vi "demux1_10(x6)_encode.vi"(8 "error in (no error)":errorcluster, 10 "demux1_10(x6)_encode":T1(ring), 11 "Mem_mapping in":u16[](array[numeric])) -> (0 "error out":errorcluster, 3 "MemMapping Out":u16[](array[numeric]))   [LabVIEW 2018, in "MB Relay.lvlib"]
uses:
  MB Relay.lvlib
panel:
  out "demux10_1(x6)":u16[](array[numeric])
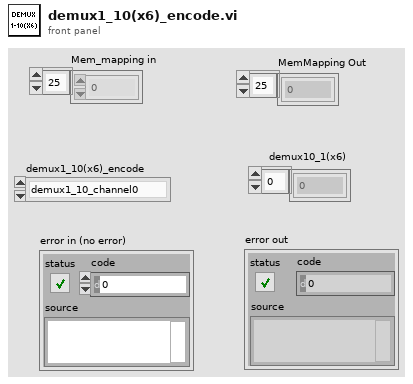
[diagram p1: front panel]
types:
  T1 = enum16{"demux1_10_channel0", "demux1_10_channel1", "demux1_10_channel2", "demux1_10_channel3", "demux1_10_channel4", "demux1_10_channel5", "demux1_10_channel6", "demux1_10_channel7", "demux1_10_channel8", "demux1_10_channel9", "demux1_10_channel10"}
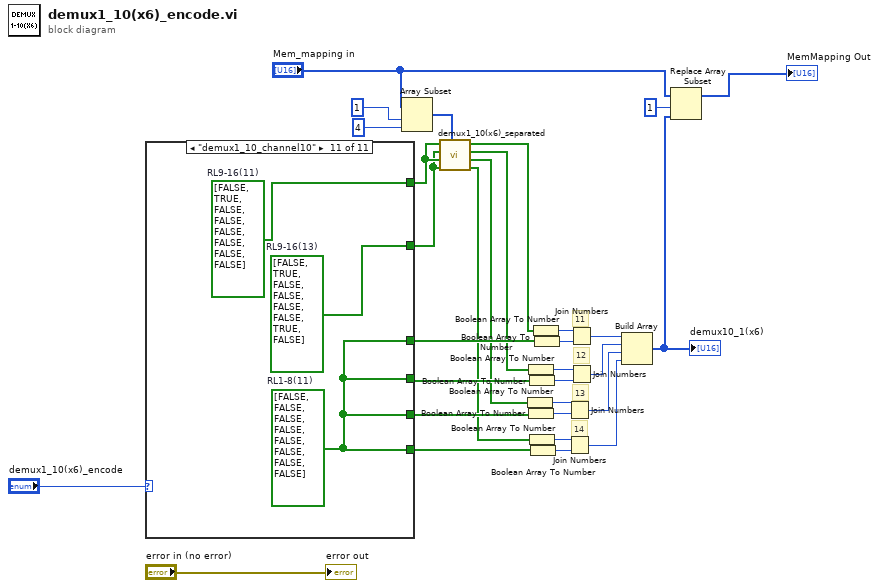
[diagram p0: block diagram]
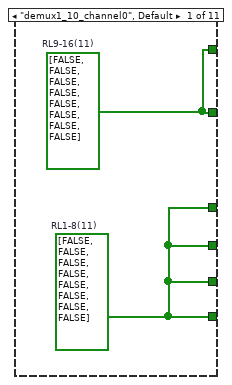
[diagram p2: hidden frame]
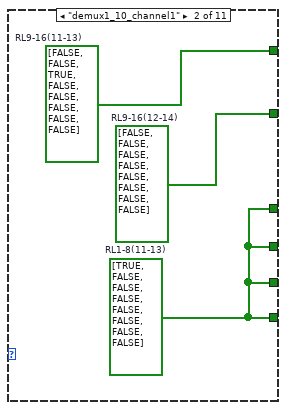
[diagram p3: hidden frame]
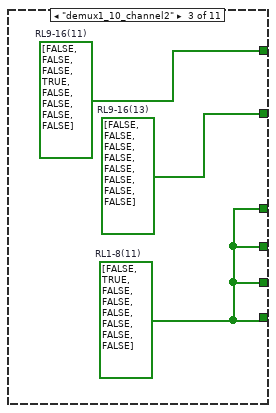
[diagram p4: hidden frame]
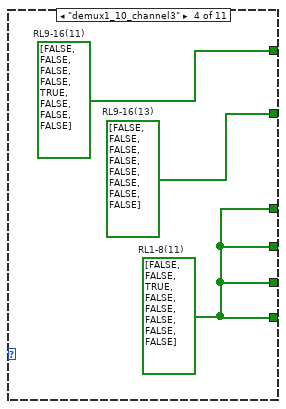
[diagram p5: hidden frame]
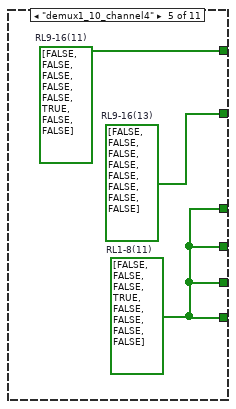
[diagram p6: hidden frame]
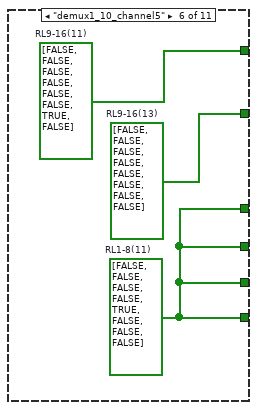
[diagram p7: hidden frame]
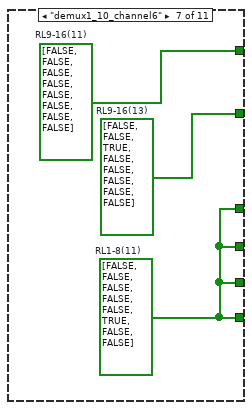
[diagram p8: hidden frame]
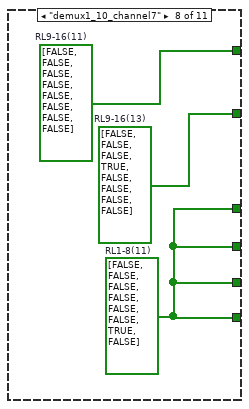
[diagram p9: hidden frame]
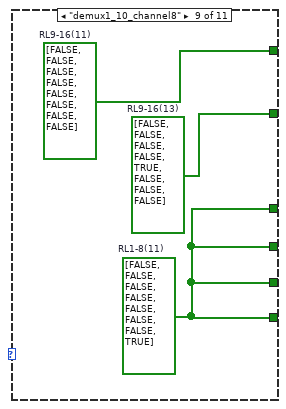
[diagram p10: hidden frame]
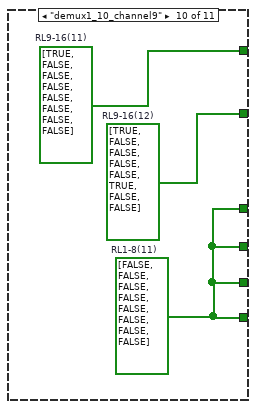
[diagram p11: hidden frame]
diagram:
  # "14"
  # "13"
  # "12"
  # "11"
  n1 = case shown="\"demux1_10_channel10\"" "demux1_10(x6)_encode" {
    tunnel: [w33 w36 w39 w42 w45 w48 w51 w54 w57 w60 w63] -> w18
    tunnel: [w33 w36 w39 w42 w45 w48 w51 w54 w57 w60 w63] -> w19
    tunnel: [w33 w36 w39 w42 w45 w48 w51 w54 w57 w60 w63] -> w17
    tunnel: [w33 w36 w39 w42 w45 w48 w51 w54 w57 w60 w63] -> w22
    tunnel: [w32 w35 w38 w41 w44 w47 w50 w53 w56 w59 w62] -> w2
    tunnel: [w32 w34 w37 w40 w43 w46 w49 w52 w55 w58 w61] -> w1
    frame "demux1_10_channel0", Default {
      w32 = bool[] [FALSE, FALSE, FALSE, FALSE, FALSE, FALSE, FALSE, FALSE]  # RL9-16(11)
      w33 = bool[] [FALSE, FALSE, FALSE, FALSE, FALSE, FALSE, FALSE, FALSE]  # RL1-8(11)
    }
    frame "demux1_10_channel1" {
      w34 = bool[] [FALSE, FALSE, FALSE, FALSE, FALSE, FALSE, FALSE, FALSE]  # RL9-16(12-14)
      w35 = bool[] [FALSE, FALSE, TRUE, FALSE, FALSE, FALSE, FALSE, FALSE]  # RL9-16(11-13)
      w36 = bool[] [TRUE, FALSE, FALSE, FALSE, FALSE, FALSE, FALSE, FALSE]  # RL1-8(11-13)
    }
    frame "demux1_10_channel2" {
      w37 = bool[] [FALSE, FALSE, FALSE, FALSE, FALSE, FALSE, FALSE, FALSE]  # RL9-16(13)
      w38 = bool[] [FALSE, FALSE, FALSE, TRUE, FALSE, FALSE, FALSE, FALSE]  # RL9-16(11)
      w39 = bool[] [FALSE, TRUE, FALSE, FALSE, FALSE, FALSE, FALSE, FALSE]  # RL1-8(11)
    }
    frame "demux1_10_channel3" {
      w40 = bool[] [FALSE, FALSE, FALSE, FALSE, FALSE, FALSE, FALSE, FALSE]  # RL9-16(13)
      w41 = bool[] [FALSE, FALSE, FALSE, FALSE, TRUE, FALSE, FALSE, FALSE]  # RL9-16(11)
      w42 = bool[] [FALSE, FALSE, TRUE, FALSE, FALSE, FALSE, FALSE, FALSE]  # RL1-8(11)
    }
    frame "demux1_10_channel4" {
      w43 = bool[] [FALSE, FALSE, FALSE, FALSE, FALSE, FALSE, FALSE, FALSE]  # RL9-16(13)
      w44 = bool[] [FALSE, FALSE, FALSE, FALSE, FALSE, TRUE, FALSE, FALSE]  # RL9-16(11)
      w45 = bool[] [FALSE, FALSE, FALSE, TRUE, FALSE, FALSE, FALSE, FALSE]  # RL1-8(11)
    }
    frame "demux1_10_channel5" {
      w46 = bool[] [FALSE, FALSE, FALSE, FALSE, FALSE, FALSE, FALSE, FALSE]  # RL9-16(13)
      w47 = bool[] [FALSE, FALSE, FALSE, FALSE, FALSE, FALSE, TRUE, FALSE]  # RL9-16(11)
      w48 = bool[] [FALSE, FALSE, FALSE, FALSE, TRUE, FALSE, FALSE, FALSE]  # RL1-8(11)
    }
    frame "demux1_10_channel6" {
      w49 = bool[] [FALSE, FALSE, TRUE, FALSE, FALSE, FALSE, FALSE, FALSE]  # RL9-16(13)
      w50 = bool[] [FALSE, FALSE, FALSE, FALSE, FALSE, FALSE, FALSE, FALSE]  # RL9-16(11)
      w51 = bool[] [FALSE, FALSE, FALSE, FALSE, FALSE, TRUE, FALSE, FALSE]  # RL1-8(11)
    }
    frame "demux1_10_channel7" {
      w52 = bool[] [FALSE, FALSE, FALSE, TRUE, FALSE, FALSE, FALSE, FALSE]  # RL9-16(13)
      w53 = bool[] [FALSE, FALSE, FALSE, FALSE, FALSE, FALSE, FALSE, FALSE]  # RL9-16(11)
      w54 = bool[] [FALSE, FALSE, FALSE, FALSE, FALSE, FALSE, TRUE, FALSE]  # RL1-8(11)
    }
    frame "demux1_10_channel8" {
      w55 = bool[] [FALSE, FALSE, FALSE, FALSE, TRUE, FALSE, FALSE, FALSE]  # RL9-16(13)
      w56 = bool[] [FALSE, FALSE, FALSE, FALSE, FALSE, FALSE, FALSE, FALSE]  # RL9-16(11)
      w57 = bool[] [FALSE, FALSE, FALSE, FALSE, FALSE, FALSE, FALSE, TRUE]  # RL1-8(11)
    }
    frame "demux1_10_channel9" {
      w58 = bool[] [TRUE, FALSE, FALSE, FALSE, FALSE, TRUE, FALSE, FALSE]  # RL9-16(12)
      w59 = bool[] [TRUE, FALSE, FALSE, FALSE, FALSE, FALSE, FALSE, FALSE]  # RL9-16(11)
      w60 = bool[] [FALSE, FALSE, FALSE, FALSE, FALSE, FALSE, FALSE, FALSE]  # RL1-8(11)
    }
    frame "demux1_10_channel10" {
      w61 = bool[] [FALSE, TRUE, FALSE, FALSE, FALSE, FALSE, TRUE, FALSE]  # RL9-16(13)
      w62 = bool[] [FALSE, TRUE, FALSE, FALSE, FALSE, FALSE, FALSE, FALSE]  # RL9-16(11)
      w63 = bool[] [FALSE, FALSE, FALSE, FALSE, FALSE, FALSE, FALSE, FALSE]  # RL1-8(11)
    }
  }
  n2 = Array Subset(array="Mem_mapping in", index=1, length=4) -> (w6:u16[])
  n3 = call "demux1_10(x6)_separated.vi"("Mem_mapping in"=w6, "Boolean array 14"=w1, "Boolean array 13"=w2, "Boolean array 12"=w1, "Boolean array 11"=w2) -> ("output array 14"=w3:bool[], "output array 13"=w4:bool[], "output array 12"=w11:bool[], "output array 11"=w5:bool[])  [unwired: 3 in]
  n4 = Boolean Array To Number(Boolean array=w4) -> (number=w15:u8)
  n5 = Boolean Array To Number(Boolean array=w11) -> (number=w16:u8)
  n6 = Boolean Array To Number(Boolean array=w19) -> (number=w14:u8)
  n7 = Boolean Array To Number(Boolean array=w17) -> (number=w20:u8)
  n8 = Boolean Array To Number(Boolean array=w3) -> (number=w13:u8)
  n9 = Boolean Array To Number(Boolean array=w18) -> (number=w12:u8)
  n10 = Boolean Array To Number(Boolean array=w5) -> (number=w23:u8)
  n11 = Boolean Array To Number(Boolean array=w22) -> (number=w21:u8)
  n12 = Join Numbers(hi=w15, lo=w14) -> ((hi.lo)=w28:u16)
  n13 = Join Numbers(hi=w13, lo=w12) -> ((hi.lo)=w29:u16)
  n14 = Join Numbers(hi=w23, lo=w21) -> ((hi.lo)=w26:u16)
  n15 = Join Numbers(hi=w16, lo=w20) -> ((hi.lo)=w27:u16)
  n16 = Build Array(w26, w27, w28, w29) -> (w9:u16[])
  "demux10_1(x6)" <- w9
  n17 = Replace Array Subset(array="Mem_mapping in", new element=w9, index=1) -> (→"MemMapping Out":u16[])
  "error out" <- "error in (no error)"
